vi "Close.vi"(8 "error in (no error)":errorcluster, 11 "session in":T1) -> (0 "error out":errorcluster)   [LabVIEW 2020, in "SLSC Switch.lvlib"]
doc: "Terminates the NI-SLSC Switch session and all of its attributes and deallocates any memory resources the driver uses."
uses:
  <vilib>/SLSC_Switch/SLSC Switch.lvlib
  nislscsl.dll
  <vilib>/userdefined/High Color/SLSC_Switch/nislscslSession.ctl
panel:
  in  "no error":errorcluster
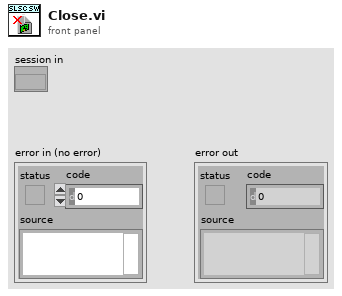
[diagram p1: front panel]
types:
  T1 = typedef "nislscslSession.ctl" = refnum<k20>
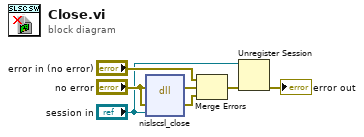
[diagram p0: block diagram]
diagram:
  n1 = dll-call lib="nislscsl.*" fn="nislscsl_close"(error in="no error", "errorCluster"="no error", "sessionHandle"="session in") -> (error out=w7:errorcluster, "errorCluster"=w6:errorcluster)  [unwired: 4 in, 1 out]
  n2 = Merge Errors("error in (no error)", w7, w6) -> (w5:errorcluster)
  n3 = Unregister Session(8:w5, 11:"session in") -> (0:→"error out":errorcluster)
